vi "Field Draw Paths.vi"(4 "Draw Targets?":T2, 6 "Lado":enum16{"Esquerdo", "Direito"}(ring), 8 "Offset":T1, 9 "Scale mm/pixel":dbl, 10 "our_robots":T3[](array[typedef]), 11 "picture in":picture) -> (3 "picture out":picture)   [LabVIEW 2017]
uses:
  Core/AI Robot.ctl
  Intel/Functions Enum.ctl
  Intel/AttackerStates.ctl
  DrawTargets.ctl
  <vilib>/Utility/miscctls.llb/LVBoundsTypeDef.ctl
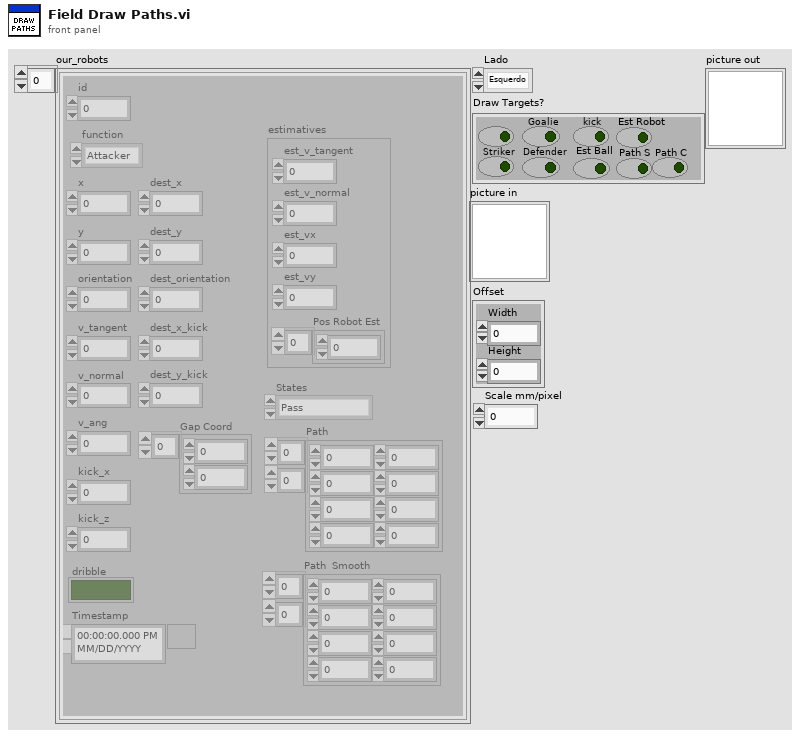
[diagram p1: front panel]
types:
  T1 = typedef "LVBoundsTypeDef.ctl" = cluster{"Width":u32, "Height":u32}
  T2 = typedef "DrawTargets.ctl" = cluster{"Attacker":bool, "Striker":bool, "Goalie":bool, "Defender":bool, "kick":bool, "Est Ball":bool, "Est Robot":bool, "Path S":bool, "Path C":bool}
  T3 = typedef "AI Robot.ctl" = cluster{"id":u32, "function":T4, "x":dbl, "y":dbl, "orientation":dbl, "v_tangent":dbl, "v_normal":dbl, "v_ang":dbl, "kick_x":dbl, "kick_z":dbl, "dribble":bool, "Timestamp":timestamp, "dest_x":dbl, "dest_y":dbl, "dest_orientation":dbl, "estimatives":cluster{"est_v_tangent":dbl, "est_v_normal":dbl, "est_vx":dbl, "est_vy":dbl, "Pos Robot Est":dbl[]}, "dest_x_kick":dbl, "dest_y_kick":dbl, "Gap Coord":dbl[], "States":T5, "Path ":dbl[][], "Path  Smooth":dbl[][]}
  T4 = typedef "Functions Enum.ctl" = enum16{"Attacker", "Goalie", "Defender", "Striker", "Goto 0", "Dummy", "Kicker", "ZigZag"}
  T5 = typedef "AttackerStates.ctl" = enum16{"Pass", "GoToTangent", "BallGetting", "GoToKick", ""}
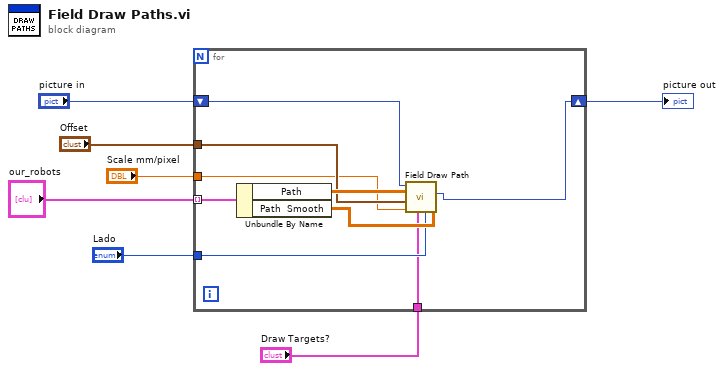
[diagram p0: block diagram]
diagram:
  n1 = for {
    tunnel: "our_robots" -> [w16] mode=indexing
    tunnel: "Lado" -> [w13]
    tunnel: "Draw Targets?" -> [w12]
    tunnel: "Offset" -> [w10]
    tunnel: "Scale mm/pixel" -> [w9]
    shift-right: [w8] -> w1
    shift-left: "picture in" -> [w11]
    n2 = Unbundle By Name(w16) -> ("Path"=w15:dbl[][], "Path  Smooth"=w14:dbl[][])
    n3 = call "Field Draw Path.vi"("Pontos Smooth"=w14, "Lado"=w13, "Draw Targets?"=w12, "Scale mm/pixel"=w9, "Offset"=w10, "Pontos"=w15, "picture in"=w11) -> ("picture out"=w8:picture)  [unwired: 4 in]
  }
  "picture out" <- w1
